vi "Configure Trigger Event Timer.vi"(0 "VISA resource name":refnum<visa-resource-name>, 1 "Trigger Count (1)":i32=1, 2 "Enable Pass Through (F: Disable)":bool, 5 "Trigger Number (1)":i32=1, 7 "Trigger Delay Type (0: Period)":i32(ring) items=["Period", "List"], 9 "Event ID":string, 11 "error in (no error)":errorcluster, 12 "Trigger Delay (1E-5 S)":dbl=1e-05, 13 "Trigger Delay List":dbl[](array[numeric])) -> (4 "VISA resource name out":refnum<visa-resource-name>, 15 "error out":errorcluster)   [LabVIEW 2019, in "Keithley 2600 Series.lvlib"]
doc: "Configures the event that triggers the timer delay.\n\n<b>Note:</b>\nIn order to allow for the configuration to achieve a known default state, it's required to call <b>Reset Trigger Event</b> VI before you call this VI."
uses:
  Keithley 2600 Series.lvlib
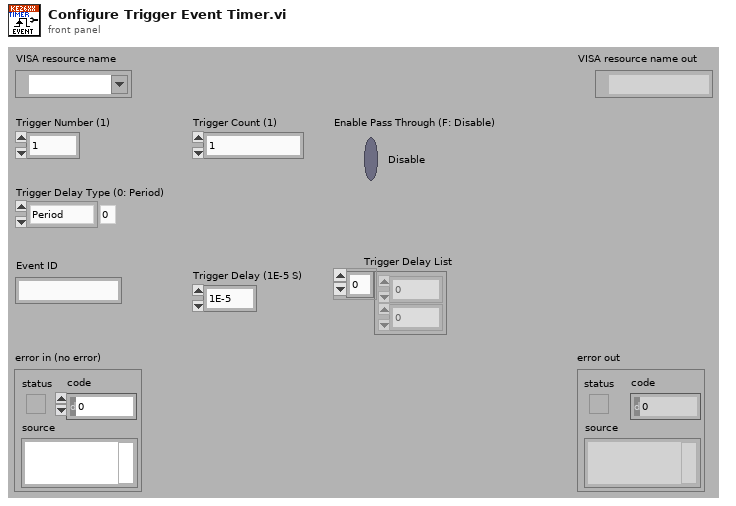
[diagram p1: front panel]
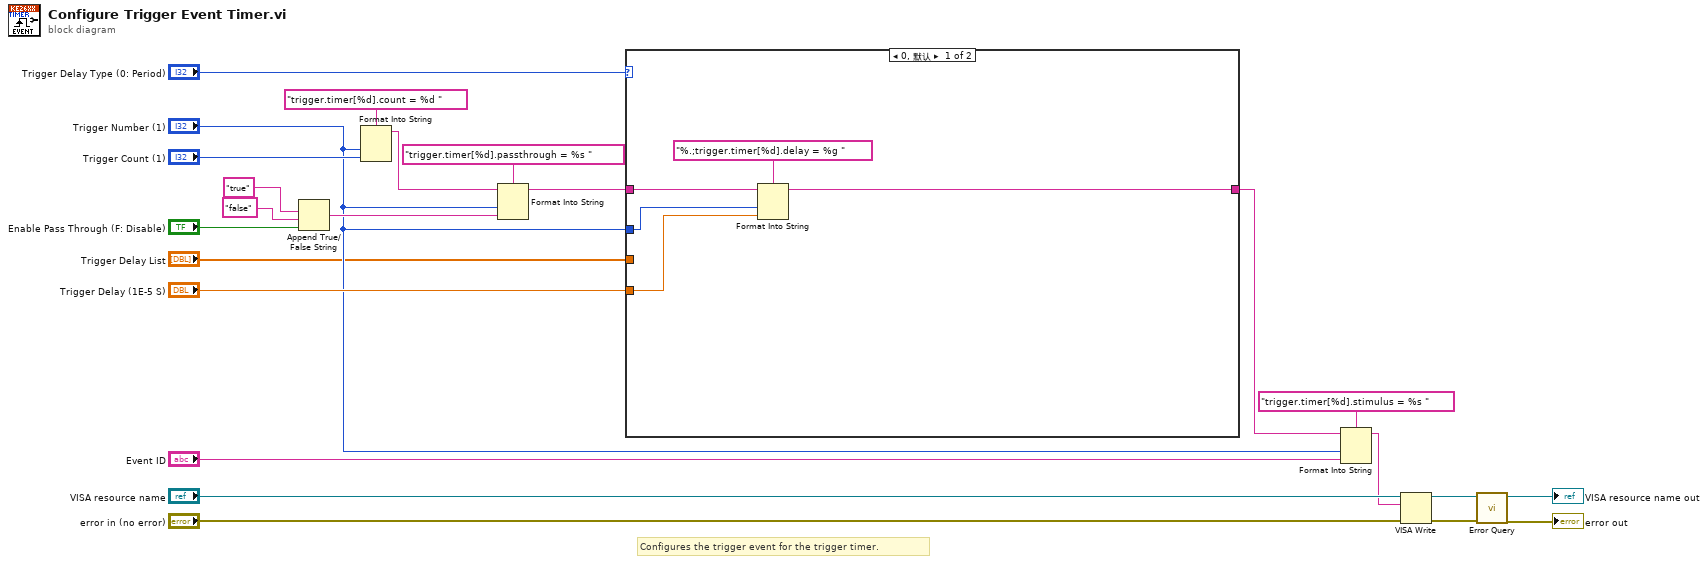
[diagram p0: block diagram]
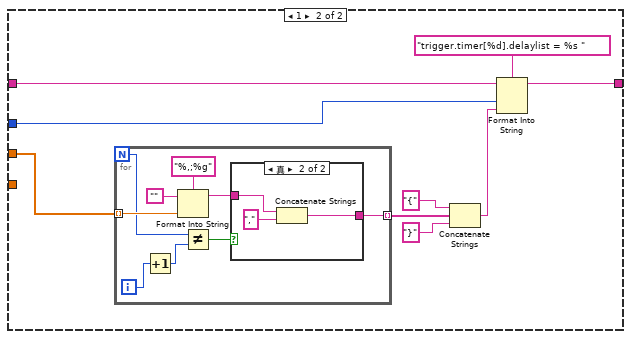
[diagram p2: hidden frame]
diagram:
  # "Configures the trigger event for the trigger timer."
  n1 = Append True/False String(1:"Enable Pass Through (F: Disable)", 2:"false", 3:"true") -> (0:w19:string)  [unwired: 1 in]
  n2 = Format Into String(format string="trigger.timer[%d].count = %d ", "Trigger Number (1)", "Trigger Count (1)") -> (resulting string=w10:string)  [unwired: 2 in, 1 out]
  n3 = Format Into String(format string="trigger.timer[%d].passthrough = %s ", initial string=w10, "Trigger Number (1)", w19) -> (resulting string=w9:string)  [unwired: 1 in, 1 out]
  n4 = case shown="0, 默认" "Trigger Delay Type (0: Period)" {
    tunnel: w9 -> [w27 w32]
    tunnel: "Trigger Number (1)" -> [w25 w31]
    tunnel: "Trigger Delay (1E-5 S)" -> [w26 _]
    tunnel: "Trigger Delay List" -> [_ w34]
    tunnel: [w24 w29] -> w6
    frame 0, Default {
      n5 = Format Into String(format string="%.;trigger.timer[%d].delay = %g ", initial string=w27, w25, w26) -> (resulting string=w24:string)  [unwired: 1 in, 1 out]
    }
    frame 1 {
      n6 = for {
        N -> [w38]
        tunnel: w34 -> [w46] mode=indexing
        tunnel: [w39] -> w37 mode=indexing
        i -> [w43]
        n7 = Increment(x=w43) -> (x+1=w42:i32)
        n8 = Format Into String(format string="%,;%g", initial string="", w46) -> (resulting string=w40:string)  [unwired: 1 in, 1 out]
        n9 = Not Equal?(x=w38, y=w42) -> (x != y?=w41:bool)
        n10 = case shown="真" w41 {
          tunnel: w40 -> [w47 w50]
          tunnel: [w47 w48] -> w39
          frame False {
          }
          frame True {
            n11 = Concatenate Strings(w50, ",") -> (w48:string)
          }
        }
      }
      n12 = Concatenate Strings("{" ("string"), w37, "}") -> (w30:string)
      n13 = Format Into String(format string="trigger.timer[%d].delaylist = %s ", initial string=w32, w31, w30) -> (resulting string=w29:string)  [unwired: 1 in, 1 out]
    }
  }
  n14 = Format Into String(format string="trigger.timer[%d].stimulus = %s ", initial string=w6, "Trigger Number (1)", "Event ID") -> (resulting string=w4:string)  [unwired: 1 in, 1 out]
  n15 = VISA Write(VISA resource name="VISA resource name", write buffer=w4, error in (no error)="error in (no error)") -> (VISA resource name out=w16:refnum<visa-resource-name>, error out=w15:errorcluster)  [unwired: 1 out]
  n16 = call "Error Query.vi"("error in (no error)"=w15, "VISA resource name"=w16) -> ("error out"=→"error out":errorcluster, "VISA resource name out"=→"VISA resource name out":refnum<visa-resource-name>)  [unwired: 6 in, 2 out]
